vi "Global SIFS.vi"() -> ()   [LabVIEW 2011]
panel:
  out "FLTR":T1
  out "RACK":T1
  out "PPULL":T1
  out "GRAT":T1
  out "SHUT":T1
  out "FOCUS":T1
  out "LENS":T1
  out "MASK":T1
  out "CAM":T1
  in  "Ppull":string[][](array[string])
  out "POS":dbl format="%#.5f"
  in  "Wave":string[][](array[string])=[["HOME", "0", "0"], ["700B", "11", "22"], ["700M", "12", "24"], ["700R", "13", "26"], ["1500M1", "13", "28"], ["1500M2", "13", "30"], ["1500M3", "13", "32"], ["1500M4", "13", "34"], ["1500M5", "13", "36"], ["2200M1", "13", "38"], ["2600M1", "13", "40"], ["3000M1", "13", "42"]]
  in  "Grating":string[][](array[string])=[["HOME", "0", "0"], ["CLEAR", "292", "0"], ["700", "292", "36"], ["1500", "292", "83"], ["2200", "292", "129"], ["2600", "292", "173"], ["3000", "292", "219"]]
  in  "Lens":string[][](array[string])=[["HOME", "0,000"], ["LENS1", "2"], ["LENS2", "82,5"]]
  in  "Mask":string[][](array[string])=[["HOME", "0,000"], ["OPEN", "106"], ["MASK0", "21,65"], ["MASK1", "22,65"], ["MASK2", "23,65"], ["MASK3", "24,65"], ["MASK4", "25,65"], ["MASK5", "26,65"], ["MASK6", "27,65"], ["MASK7", "28,65"]]
  in  "Filter":string[][](array[string])=[["HOME", "0,000"], ["SBIG", "3,35"], ["CLEAR", "31,5"], ["FILTER1", "32,5"], ["FILTER2", "33,5"], ["FILTER3", "34,5"]]
  # "cam-angle"
  # "gr-angle"
  # "push-pull"
  # "rack"
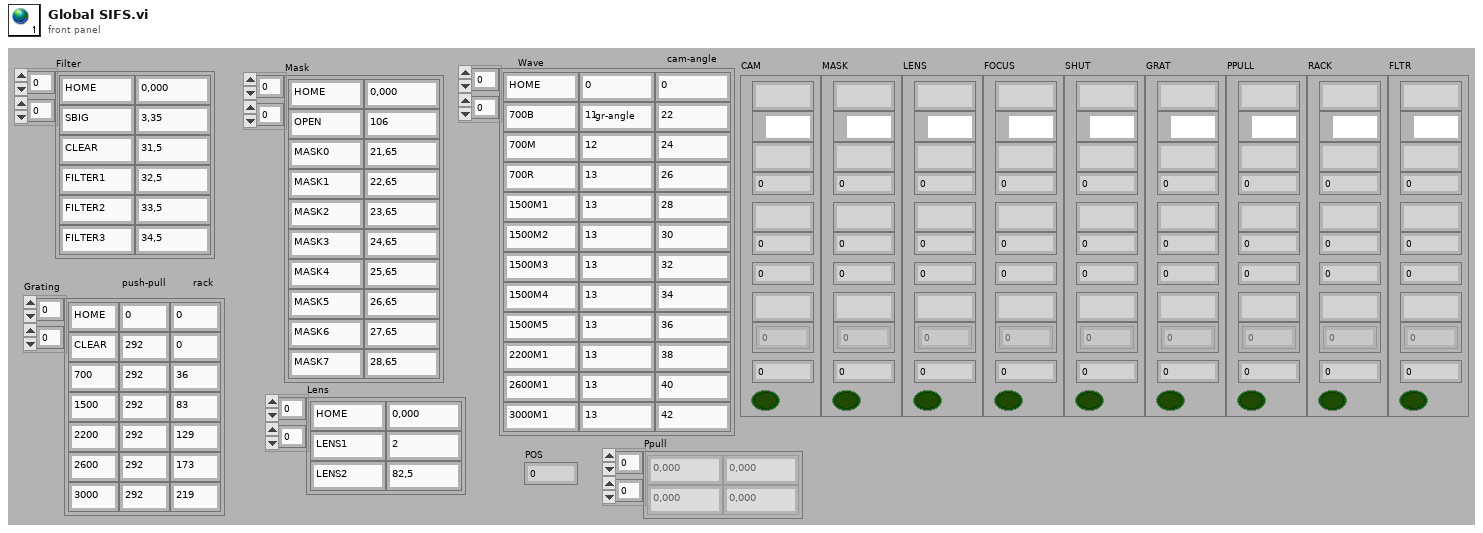
[diagram p1: front panel]
types:
  T1 = cluster{"Mec ID":string, "VISA Mec":refnum<visa-resource-name>, "Mec PosLimit":string, "Mec NegLimit":string, "Mec Factor":dbl, "Mec Speed":dbl, "Mec Acceleration":dbl, "MecOffset":string, "MecTargets":dbl[], "MecEnabled":bool, "Mec Target":dbl}
diagram:
